vi "week06_Ex02.vi"() -> ()   [LabVIEW 2017]
panel:
  out "String":string
  in  "Numeric":i32
  out "i":i32
  out "i-1":dbl
  out "i-2":dbl
  out "x+y":dbl
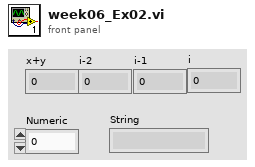
[diagram p1: front panel]
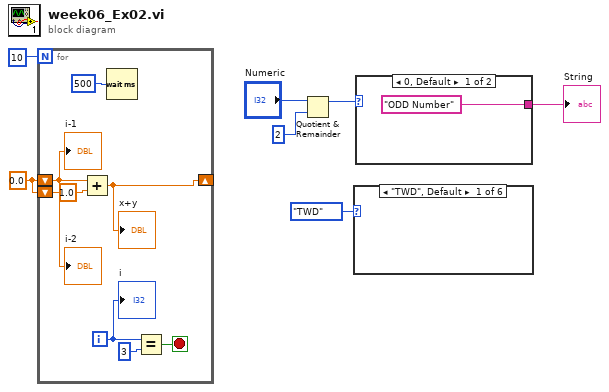
[diagram p0: block diagram]
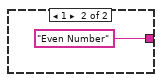
[diagram p7: hidden frame]
diagram:
  w6 = 0.0
  n1 = for {
    N: 10 -> [_]
    shift-right: [w13] -> _
    shift-left: w6 -> [w15]
    shift-left: w6 -> [w11]
    i -> [w8]
    stop <- w9 stop-if-true
    n2 = Add(x=w15, y=1.0) -> (x+y=w13:dbl)
    "x+y" <- w13
    n3 = Wait (ms)(milliseconds to wait=u32 500) -> ()  [unwired: 1 out]
    n4 = Equal?(x=w8, y=3) -> (x = y?=w9:bool)
    "i-2" <- w11
    "i-1" <- w15
    "i" <- w8
  }
  n5 = Quotient & Remainder(x="Numeric", y=2) -> (x-y*floor(x/y)=w2:i32)  [unwired: 1 out]
  n6 = case shown="\"TWD\", Default" enum16{"TWD", "US", "THB", "JPY", "EUR", ""}."TWD" {
    frame "TWD", Default {
    }
    frame "US" {
    }
    frame "THB" {
    }
    frame "JPY" {
    }
    frame "EUR" {
    }
    frame "" {
    }
  }
  n7 = case shown="0, Default" w2 {
    tunnel: ["ODD Number" "Even Number"] -> w5
    frame 0, Default {
    }
    frame 1 {
    }
  }
  "String" <- w5
